vi "Resize And Position FP.vi"(8 "error in (no error)":errorcluster, 11 "VI Reference":refnum<vi>) -> (0 "error out":errorcluster, 3 "VI Reference out":refnum<vi>)   [LabVIEW 2020, in "Choose Implementation Dialog.lvlib"]
uses:
  <resource>/dialog/lvconfig.llb/LV Config Read String.vi
  Choose Implementation Dialog.lvlib
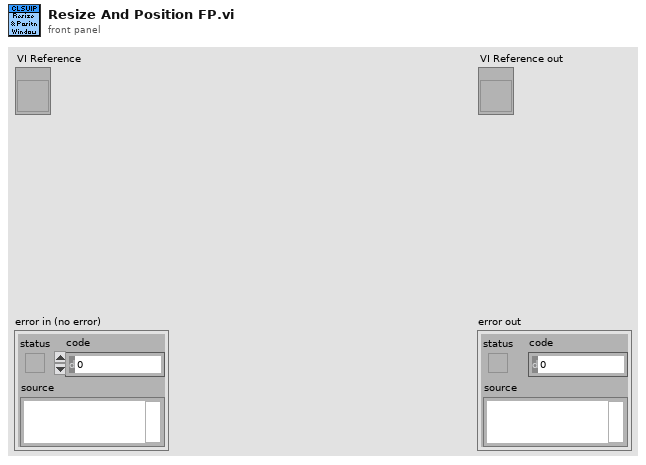
[diagram p1: front panel]
types:
  T1 = cluster{"left":i16, "top":i16, "right":i16, "bottom":i16}
  T2 = typedef "LVRectTypeDef.ctl" = cluster{"Left":i16, "Top":i16, "Right":i16, "Bottom":i16}
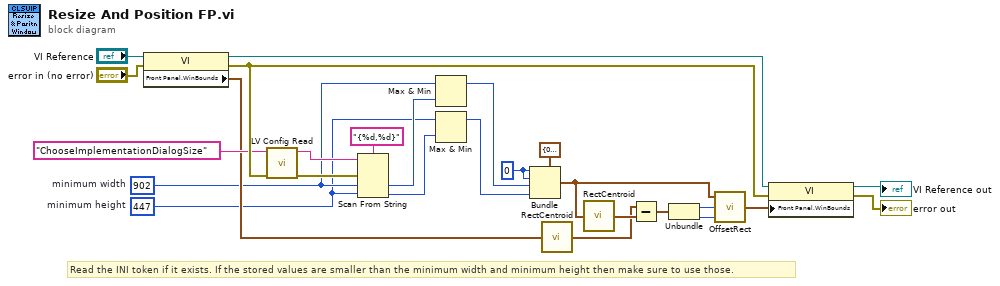
[diagram p0: block diagram]
diagram:
  w15 = i16 0 ("y")
  w3 = i16 447  # minimum height
  w6 = i16 902  # minimum width
  # "Read the INI token if it exists. If the stored values are smaller than the minimum width and minimum height then make sure to use those."
  n1 = property class="VI"(reference="VI Reference", error in="error in (no error)") -> (reference out=w22:refnum<vi>, error out=w20:errorcluster, "Front Panel.WinBounds"=w14:T2)
  n2 = call-poly <resource>:"LV Config Read.vi"("error in"=w20, "key"="ChooseImplementationDialogSize" ("Name")) -> ("error out"=w17:errorcluster, "value"=w18:string)  [unwired: 3 in, 1 out]
  n3 = Scan From String(format string="{%d,%d}", input string=w18, error in=w17, default 1=w6, default 2=w3) -> (output 1=w5:i16, output 2=w2:i16)  [unwired: 1 in, 3 out]
  n4 = Max & Min(x=w6, y=w5) -> (max(x,y)=w4:i16)  [unwired: 1 out]
  n5 = Max & Min(x=w3, y=w2) -> (max(x,y)=w1:i16)  [unwired: 1 out]
  n6 = Bundle(cluster=T1 {"left"=0, "top"=0, "right"=0, "bottom"=0} ("offset rect"), "left"=w15, "top"=w15, "right"=w4, "bottom"=w1) -> (w10:T1)
  n7 = call <vilib>:"RectCentroid.vi"("rect"=w14) -> ("point"=w12:cluster{"x":i16, "y":i16})
  n8 = call <vilib>:"RectCentroid.vi"("rect"=w10) -> ("point"=w13:cluster{"x":i16, "y":i16})
  n9 = Subtract(x=w12, y=w13) -> (x-y=w11:cluster{"x":i16, "y":i16})
  n10 = Unbundle(w11) -> ("x"=w9:i16, "y"=w8:i16)
  n11 = call <vilib>:"OffsetRect.vi"("v"=w8, "h"=w9, "rect"=w10) -> ("offset rect"=w7:T1)
  n12 = property class="VI"(reference=w22, error in=w20, "Front Panel.WinBounds"=w7) -> (reference out=→"VI Reference out":refnum<vi>, error out=→"error out":errorcluster)
